vi "condAmbientalesIniciales.vi"(8 "error in (no error)":errorcluster, 11 "Sonometro in":refnum<class "Sonometro.lvclass">) -> (0 "error out":errorcluster, 3 "Sonometro out":refnum<class "Sonometro.lvclass">)   [LabVIEW 2019, in "Sonometro.lvclass"]
uses:
  Sonometro.lvclass
  Base de Datos/SQLiteConnector/SQLiteConnection.lvclass
  Base de Datos/Base de Datos.lvclass
panel:
  out "humedad_ok":bool
  out "presion_ok":bool
  out "temp_ok":bool
  out "humedad_corregida":dbl
  out "presion_corregida":dbl
  out "temp_corregida":dbl
  in  "salir":bool
  in  "humedad":dbl
  in  "presion":dbl
  in  "temperatura":dbl
  # "Medido"
  # "Corregido"
  # "Cumple"
  # "Humedad [%]"
  # "Presión [hPa]"
  # "Temperatura [°C]"
  # "Condiciones Ambientales \nINICIALES"
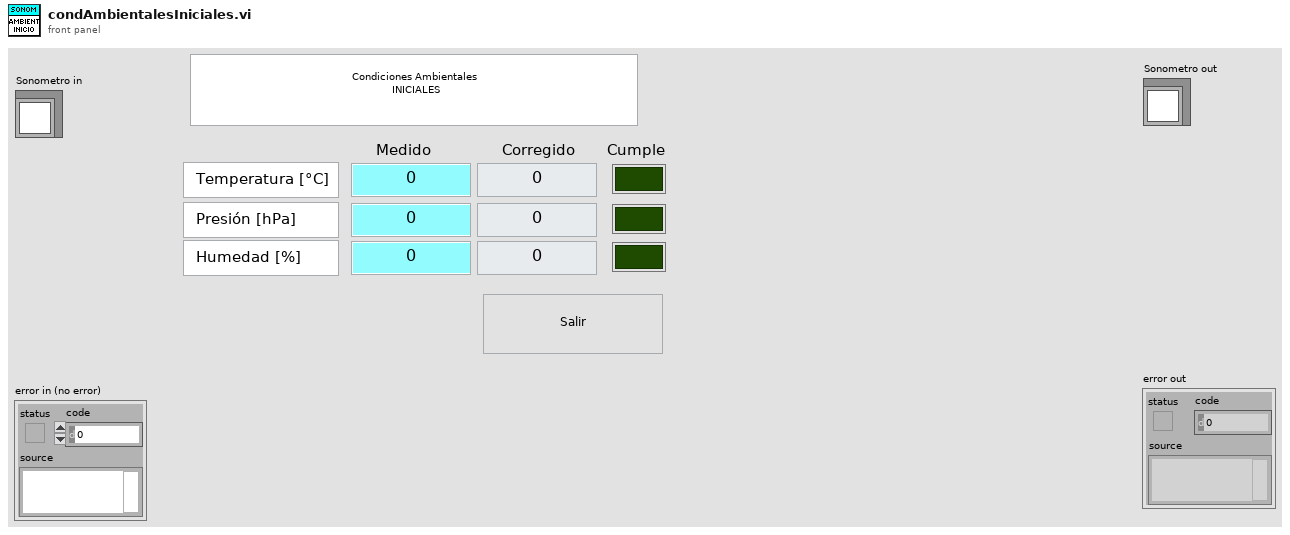
[diagram p1: front panel]
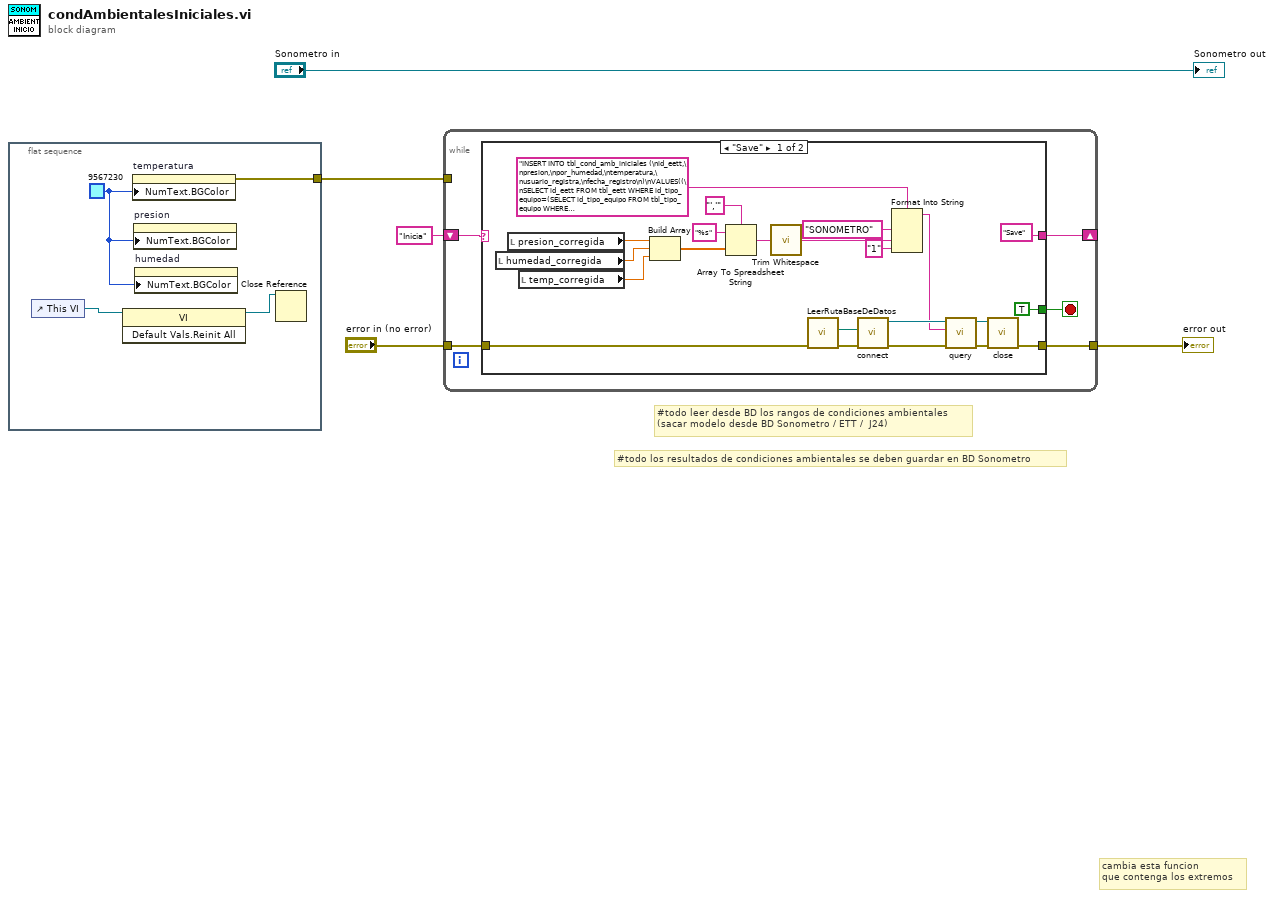
[diagram p0: block diagram]
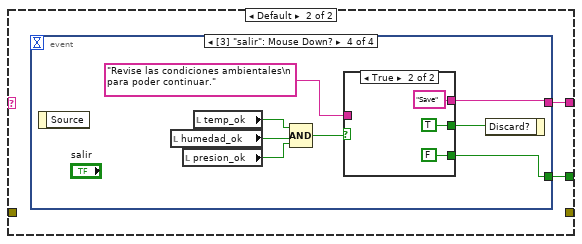
[diagram p2: hidden frame]
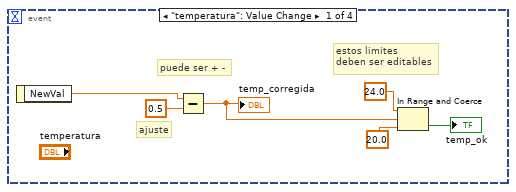
[diagram p3: hidden frame]
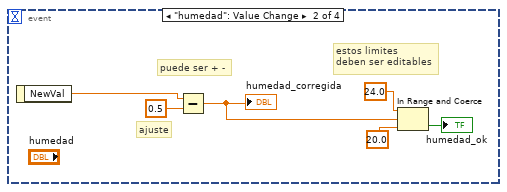
[diagram p4: hidden frame]
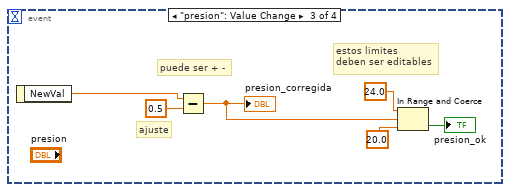
[diagram p5: hidden frame]
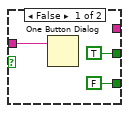
[diagram p6: hidden frame]
diagram:
  # "#todo los resultados de condiciones ambientales se deben guardar en BD Sonometro"
  # "cambia esta funcion\nque contenga los extremos"
  # "#todo leer desde BD los rangos de condiciones ambientales\n(sacar modelo desde BD Sonometro / ETT /  J24)"
  n1 = flat-sequence {
    tunnel: [w8] -> w4
    frame #0 {
      w9 = u32 9567230
      n2 = control-ref of="This VI"() -> (w7:refnum<vi>)
      n3 = invoke class="VI" method="Default Vals.Reinit All"(reference=w7) -> (reference out=w6:refnum<vi>)  [unwired: 2 in, 2 out]
      n4 = property on="temperatura" class="DigNum (strict)"("NumText.BGColor"=w9) -> (error out=w8:errorcluster)  [unwired: 2 in, 1 out]
      n5 = property on="presion" class="DigNum (strict)"("NumText.BGColor"=w9) -> ()  [unwired: 2 in, 2 out]
      n6 = property on="humedad" class="DigNum (strict)"("NumText.BGColor"=w9) -> ()  [unwired: 2 in, 2 out]
      n7 = Close Reference(reference=w6) -> ()  [unwired: 1 in, 1 out]
    }
  }
  n8 = while {
    tunnel: w4 -> [_]
    shift-right: [w12] -> _
    shift-left: "Inicia" -> [w13]
    tunnel: [w11] -> w2
    tunnel: "error in (no error)" -> [w10]
    stop <- w14 stop-if-true
    n9 = case shown="\"Save\"" w13 {
      tunnel: [TRUE w38] -> w14
      tunnel: ["Save" w37] -> w12
      tunnel: [w16 _] -> w11
      tunnel: w10 -> [w15 _]
      frame "Save" {
        n10 = local read "humedad_corregida"() -> (w25:dbl)
        n11 = local read "presion_corregida"() -> (w24:dbl)
        n12 = local read "temp_corregida"() -> (w26:dbl)
        n13 = Build Array(w24, w25, w26) -> (w23:dbl[])
        n14 = Array To Spreadsheet String(delimiter (Tab)="','", array=w23, 3:"%s" ("format string")) -> (spreadsheet string=w19:string)
        n15 = call <vilib>:"Trim Whitespace.vi"("string"=w19) -> ("trimmed string"=w18:string)  [unwired: 1 in]
        n16 = call "LeerRutaBaseDeDatos.vi"("error in (no error)"=w15) -> ("error out"=w29:errorcluster, "Database Path"=w30:path)  [unwired: 9 in]
        n17 = call "connect.vi"("error in (no error)"=w29, "Database Path"=w30) -> ("error out"=w32:errorcluster, "object out"=w31:refnum<class "SQLiteConnection.lvclass">)  [unwired: 8 in]
        n18 = Format Into String(format string="INSERT INTO tbl_cond_amb_iniciales (\nid_eett,\npresion,\npor_humedad,\ntemperatura,\nusuario_registra,\nfecha_registro\n)\nVALUES((\nSELECT id_eett FROM tbl_eett WHERE id_tipo_equipo=(SELECT id_tipo_equipo FROM tbl_tipo_equipo WHERE nombre='%s')),'%s','%s',DATETIME('NOW'))" ("SQL Statement"), "SONOMETRO" ("input 1"), w18, "1" ("input 2")) -> (resulting string=w27:string)  [unwired: 2 in, 1 out]
        n19 = call "query.vi"("error in (no error)"=w32, "SQL Statement"=w27, "object in"=w31) -> ("error out"=w34:errorcluster, "object out"=w33:refnum<class "SQLiteConnection.lvclass">)  [unwired: 5 in, 2 out]
        n20 = call-dynamic "close.vi"("error in (no error)"=w34, "object in"=w33) -> ("error out"=w16:errorcluster)  [unwired: 8 in, 1 out]
      }
      frame Default {
        n21 = event shown="[3] \"salir\": Mouse Down?" {
          selector: _ -> [_ _ _ _]
          dyn-events: _ -> [_ _ _ _]
          timeout: _ -> [_ _ _ _]
          tunnel: [_ _ _ w58] -> w38
          tunnel: [_ _ _ w57] -> w37
          event "temperatura": Value Change {
            # "estos limites\ndeben ser editables"
            # "puede ser + -"
            # "ajuste"
            n22 = event-data() -> ("NewVal"=w39:dbl)  [unwired: 1 in]
            n23 = Subtract(x=w39, y=0.5) -> (x-y=w44:dbl)
            "temp_corregida" <- w44
            n24 = In Range and Coerce(upper limit=24.0, x=w44, lower limit=20.0) -> (In Range?=→"temp_ok":bool)  [unwired: 1 out]
          }
          event "humedad": Value Change {
            # "estos limites\ndeben ser editables"
            # "puede ser + -"
            # "ajuste"
            n25 = event-data() -> ("NewVal"=w47:dbl)  [unwired: 1 in]
            n26 = Subtract(x=w47, y=0.5) -> (x-y=w46:dbl)
            "humedad_corregida" <- w46
            n27 = In Range and Coerce(upper limit=24.0, x=w46, lower limit=20.0) -> (In Range?=→"humedad_ok":bool)  [unwired: 1 out]
          }
          event "presion": Value Change {
            # "estos limites\ndeben ser editables"
            # "puede ser + -"
            # "ajuste"
            n28 = event-data() -> ("NewVal"=w53:dbl)  [unwired: 1 in]
            n29 = Subtract(x=w53, y=0.5) -> (x-y=w52:dbl)
            "presion_corregida" <- w52
            n30 = In Range and Coerce(upper limit=24.0, x=w52, lower limit=20.0) -> (In Range?=→"presion_ok":bool)  [unwired: 1 out]
          }
          event "salir": Mouse Down? {
            n31 = event-data() -> ()  [unwired: 1 in, 1 out]
            n32 = local read "humedad_ok"() -> (w63:bool)
            n33 = local read "presion_ok"() -> (w62:bool)
            n34 = local read "temp_ok"() -> (w64:bool)
            n35 = Compound Arithmetic op=AND(w64, w63, w62) -> (w61:bool)
            n36 = case shown="True" w61 {
              tunnel: "Revise las condiciones ambientales\n           para poder continuar." -> [w67 _]
              tunnel: [TRUE TRUE] -> w59
              tunnel: [FALSE FALSE] -> w58
              tunnel: [_ "Save"] -> w57
              frame False {
                n37 = One Button Dialog(message=w67) -> ()  [unwired: 1 in, 1 out]
              }
              frame True {
              }
            }
            n38 = event-data("Discard?"=w59) -> ()  [unwired: 1 in, 1 out]
          }
        }
      }
    }
  }
  "error out" <- w2
  "Sonometro out" <- "Sonometro in"
